vi "PQsendQueryParams.vi"(0 "conn":u32, 1 "command":string, 2 "nParams":u32, 3 "paramTypes":u32, 4 "paramValues":u8[](array[numeric]), 5 "paramLengths":u32, 7 "paramFormats":u32, 9 "resultFormat":u32, 11 "error in (no error)":errorcluster) -> (15 "PQsendQueryParams":u32, 18 "error out":errorcluster)   [LabVIEW 2019, in "libpqlv.lvlib"]
doc: "http://www.postgresql.org/docs/8.3/static/libpq-async.html"
uses:
  libpqlv.lvlib
  libpq.dll
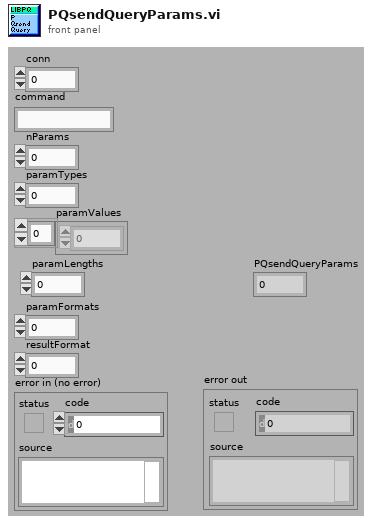
[diagram p1: front panel]
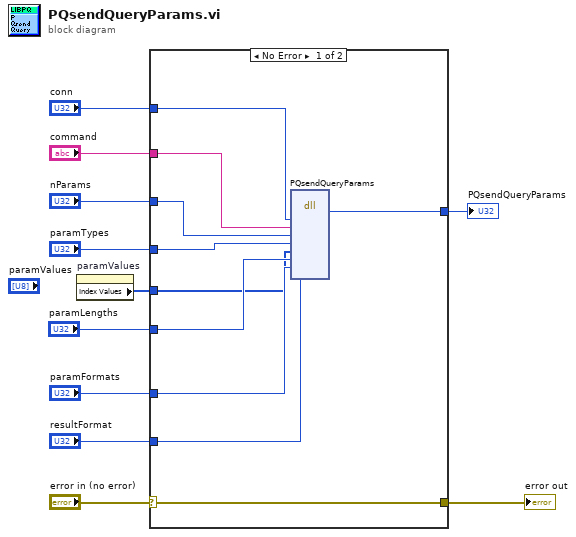
[diagram p0: block diagram]
diagram:
  n1 = property on="paramValues" class="Arr (strict)"() -> ("Index Values"=w1:u32[])  [unwired: 2 in, 2 out]
  n2 = case shown="No Error" "error in (no error)" {
    selector: "error in (no error)" -> [w21 w22]
    tunnel: [w21 w22] -> w10
    tunnel: [w20 _] -> w9
    tunnel: "command" -> [w19 _]
    tunnel: "nParams" -> [w18 _]
    tunnel: "paramTypes" -> [w17 _]
    tunnel: "paramFormats" -> [w16 _]
    tunnel: "resultFormat" -> [w15 _]
    tunnel: "conn" -> [w14 _]
    tunnel: "paramLengths" -> [w13 _]
    tunnel: w1 -> [w12 _]
    frame No Error {
      n3 = dll-call lib="libpq.*" fn="PQsendQueryParams"("conn"=w14, "command"=w19, "nParams"=w18, "paramTypes"=w17, "paramValues"=w12, "paramLengths"=w13, "paramFormats"=w16, "resultFormat"=w15) -> ("PQsendQueryParams"=w20:u32)  [unwired: 11 in, 2 out]
    }
    frame Error {
    }
  }
  "PQsendQueryParams" <- w9
  "error out" <- w10
